vi "CalculatorMain.vi"(0 "Operations Combo Box":string(combo)="Add", 1 "Load":bool, 5 "Add":bool, 7 "Delete":bool, 9 "Save":bool, 11 "error in":errorcluster, 12 "Tree":string(tree)) -> (15 "error out":errorcluster)   [LabVIEW 2023]
doc: "This is a simple calculator which can perform basic arithmetic operations like add, subtract, multiply and divide."
uses:
  Typedef/ClassClusters.ctl
  Arithmetic/Arithmetic.lvclass
  Typedef/InstancesArray.ctl
  Typedef/DVRcluster.ctl
  Typedef/DVRInstances.ctl
  Typedef/OperationsCluster.ctl
  Typedef/QueueOperations.ctl
  e65ca531-41e1-4409-bf9f-30391f5100e7.vi
  e245d3c5-e7f7-4b04-94a4-c7f52ab5977d.vi
  <vilib>/Utility/xml.llb/Write to XML File(string).vi
  <vilib>/Utility/xml.llb/Read From XML File(array).vi
panel:
  # "CALCULATOR"
  # "INSTRUCTIONS\n\n1. Run the VI.\n2. Choose the operations to perform from the Operations Combo Box.\n3. Press ADD to display once instance of the operations in the Tree.\n4. Press any instances in the tree to load that particular operations in \n    the subpanel.\n5. In the Sub-panel enter the inputs and press CALCULATE to get the \n     output.\n6. Press SAVE to save the operations data in the XML file.\n7. Press LOAD to retrive the save data from the XML, and press the saved\n    instance in the tree to display in the subpanel.\n8. Select any instance and press DELETE to reove from the tree.\n9. Close the Front panel to abort the VI."
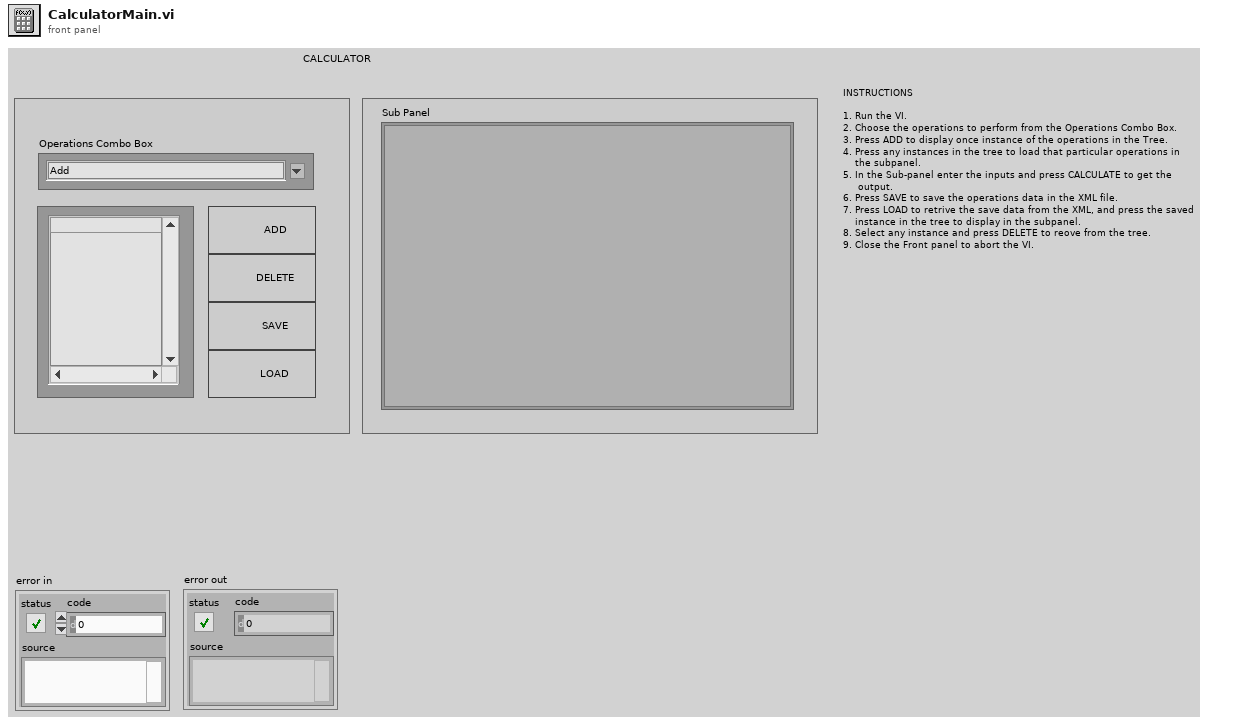
[diagram p1: front panel]
types:
  T1 = typedef "QueueOperations.ctl" = enum16{"Create", "Enqueue", "Enqueue N elements", "Dequeue", "Flush", "Release"}
  T2 = typedef "ClassClusters.ctl" = cluster{"Check":bool, "Combo Box":string, "Add":bool, "Delete":bool, "Path":path, "Tag":string, "Operation data":refnum<class "Arithmetic.lvclass">, "Instances Array":T3[], "XML path":path, "DVR":T4, "Operations Data":T6, "Saved Instances":string[], "Saves Instances String":string, "Saved Instances Path":path, "Class Path":path}
  T3 = typedef "InstancesArray.ctl" = cluster{"Tag":string, "Operation data":refnum<class "Arithmetic.lvclass">}
  T4 = typedef "DVRcluster.ctl" = cluster{"data value reference out":refnum<data-value>, "Operation Data DVR":refnum<data-value>, "Instances Array DVR":T5[]}
  T5 = typedef "DVRInstances.ctl" = cluster{"Operation Data DVR":refnum<data-value>, "Tag":string}
  T6 = typedef "OperationsCluster.ctl" = cluster{"A":dbl, "B":dbl, "C":dbl}
  T7 = typedef "LVPoint32TypeDef.ctl" = cluster{"Horizontal":i32, "Vertical":i32}
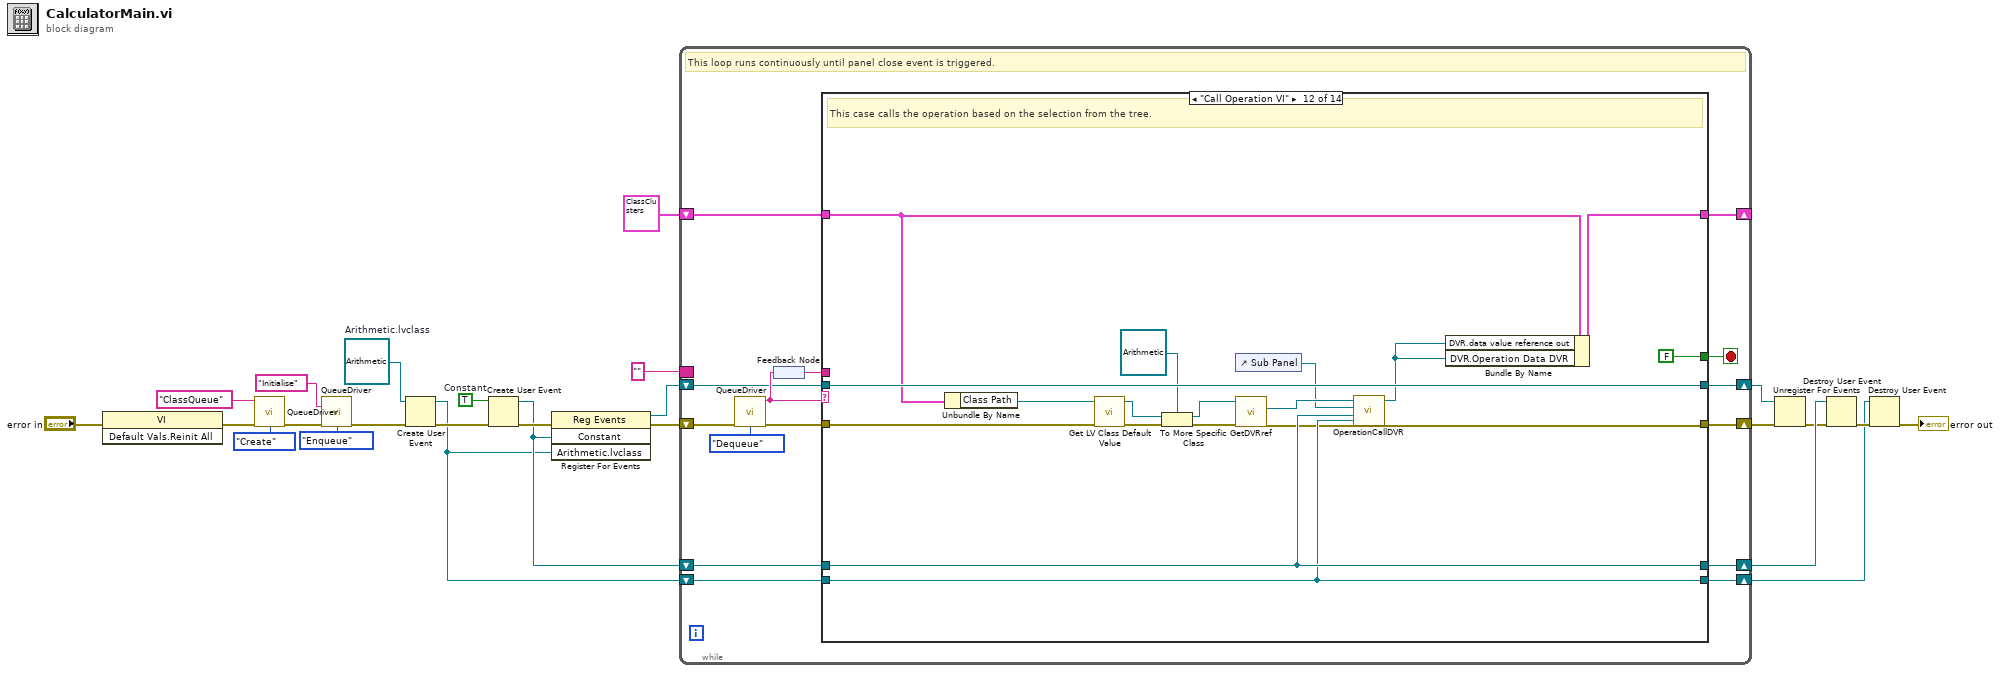
[diagram p0: block diagram]
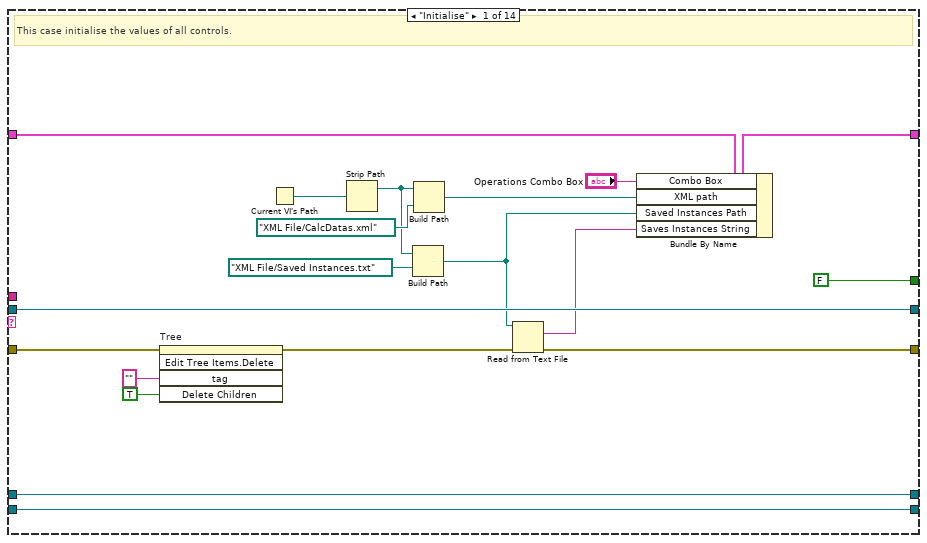
[diagram p2: hidden frame]
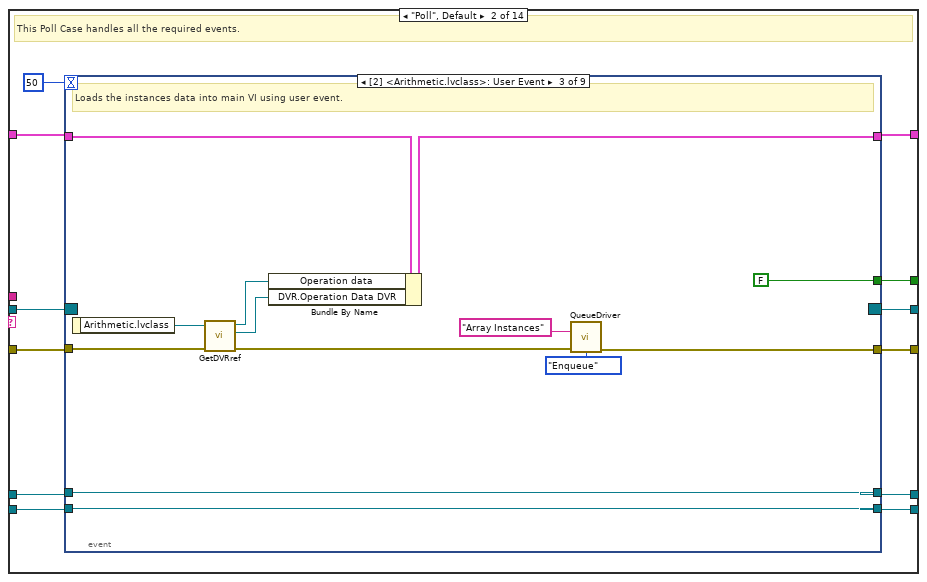
[diagram p3: hidden frame]
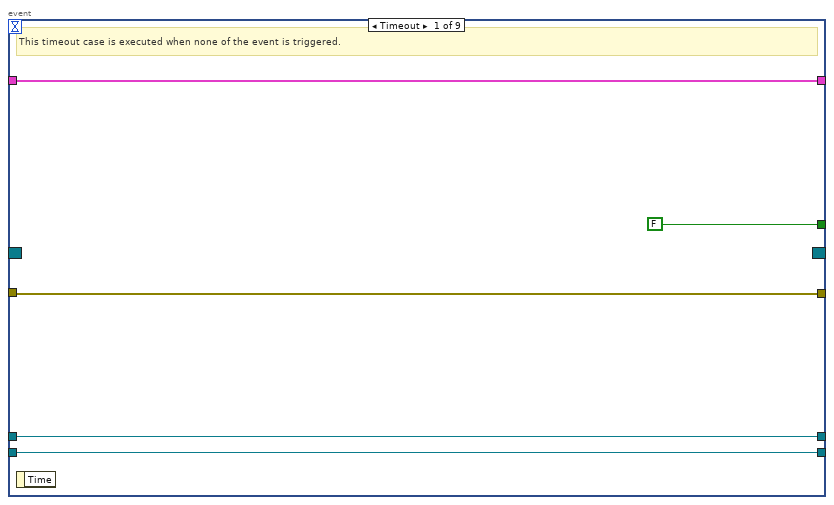
[diagram p4: hidden frame]
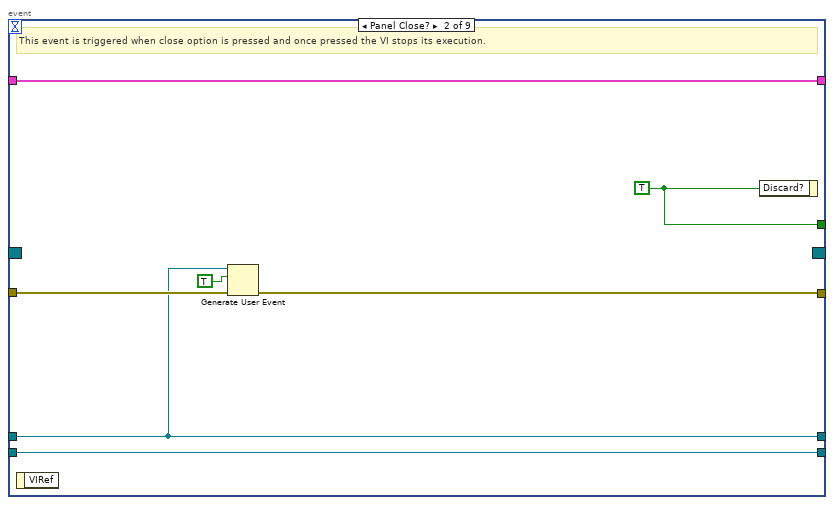
[diagram p5: hidden frame]
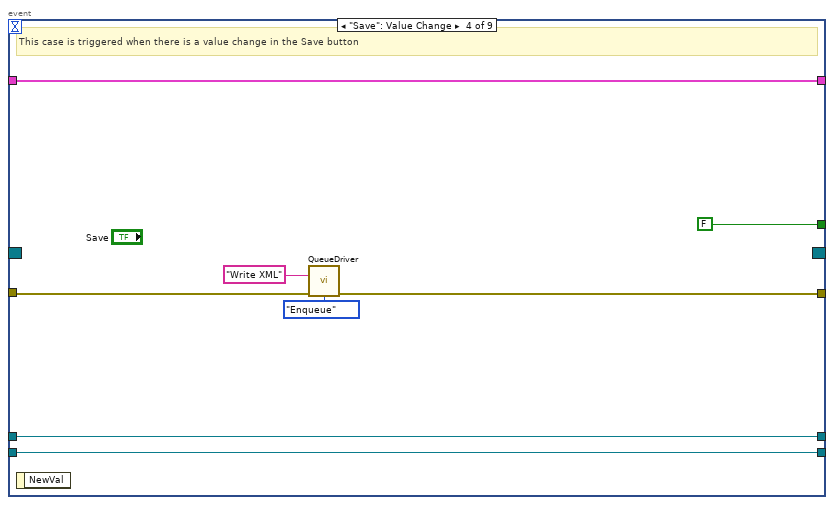
[diagram p6: hidden frame]
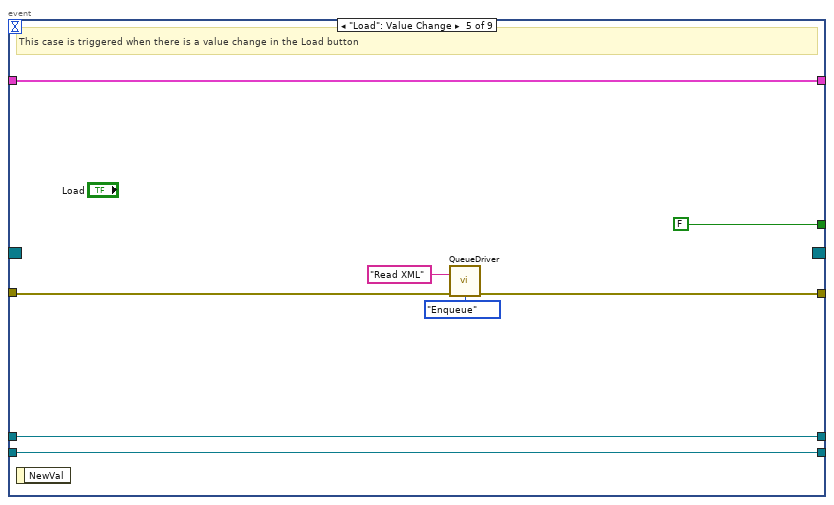
[diagram p7: hidden frame]
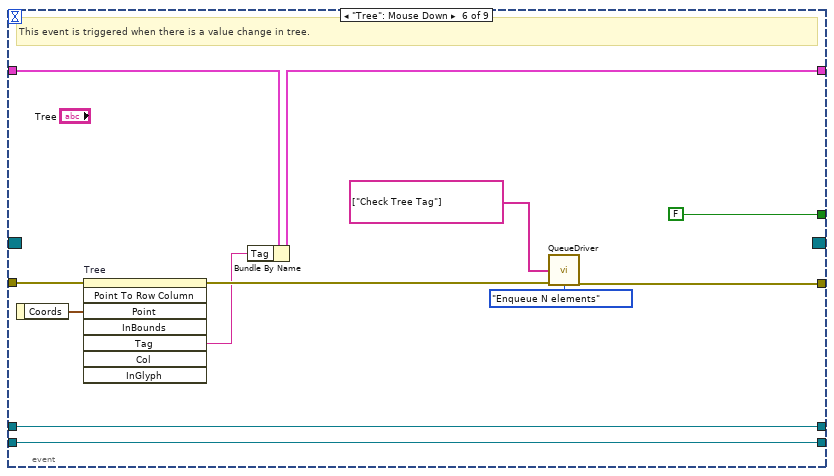
[diagram p8: hidden frame]
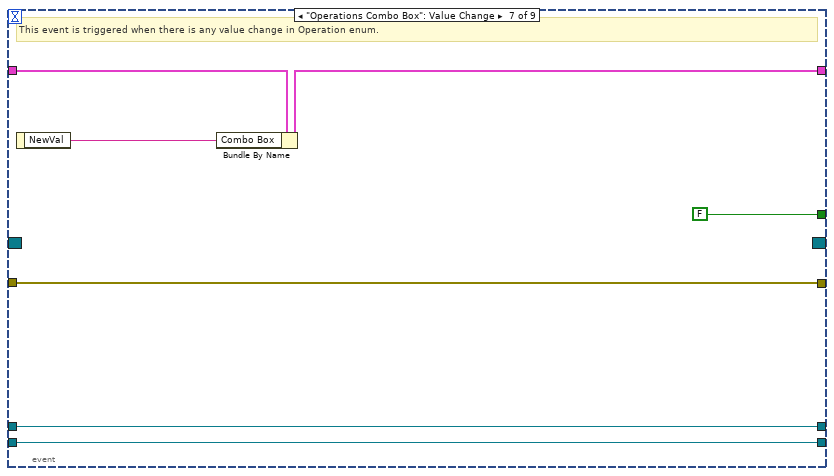
[diagram p9: hidden frame]
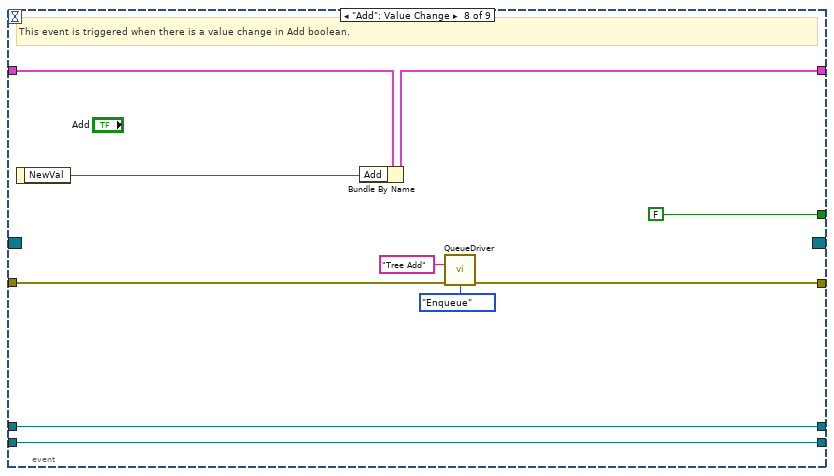
[diagram p10: hidden frame]
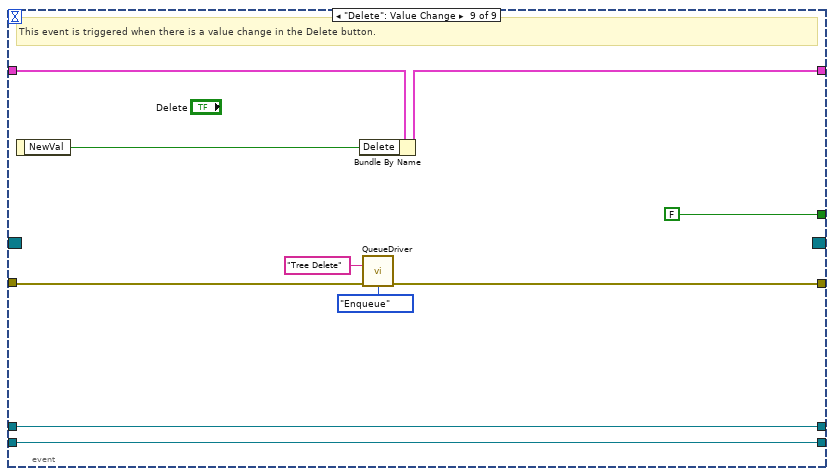
[diagram p11: hidden frame]
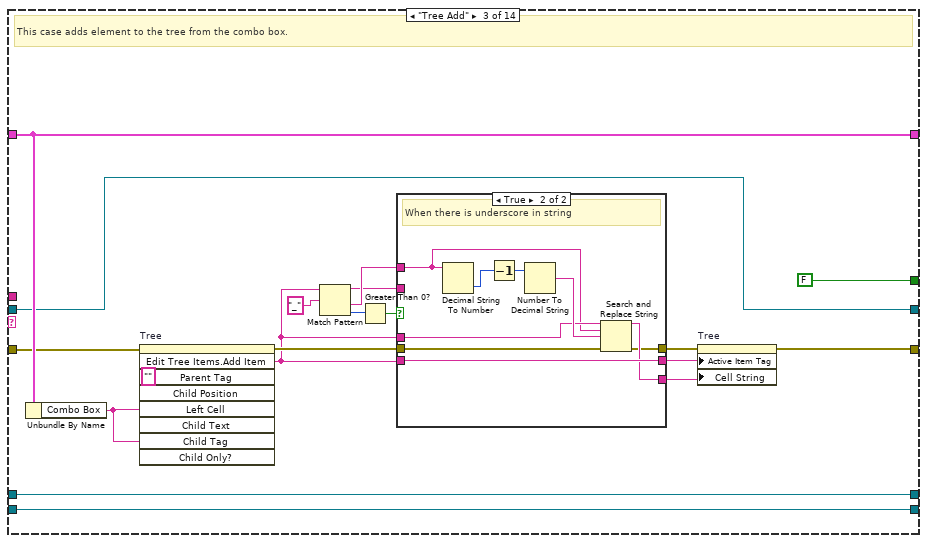
[diagram p12: hidden frame]
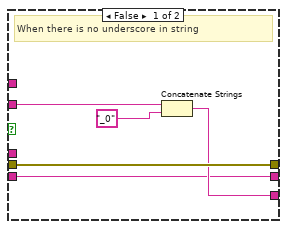
[diagram p13: hidden frame]
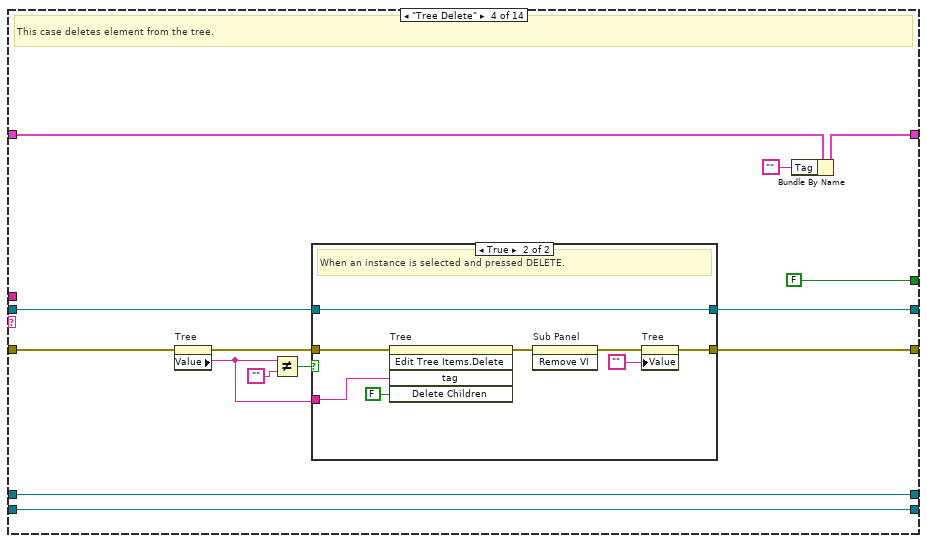
[diagram p14: hidden frame]
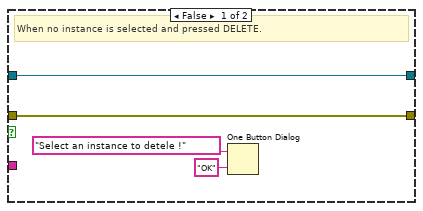
[diagram p15: hidden frame]
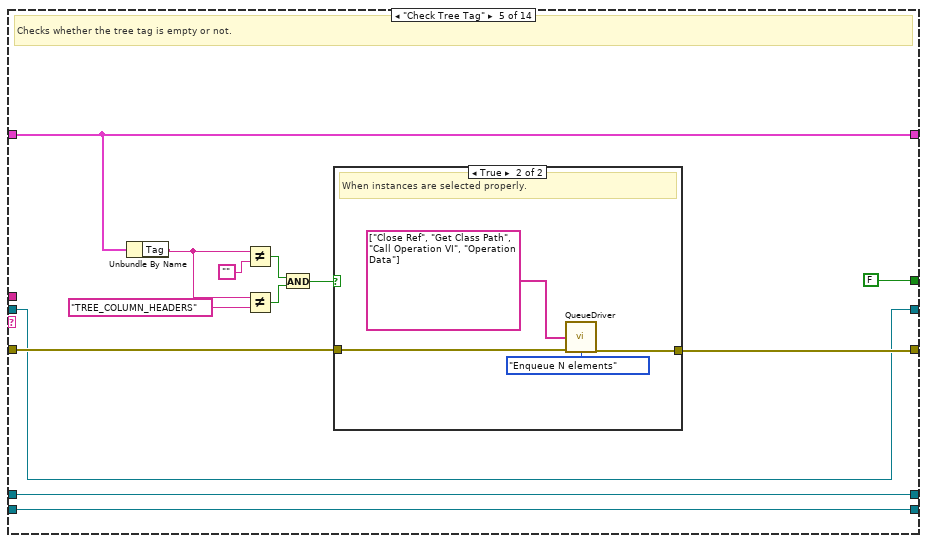
[diagram p16: hidden frame]
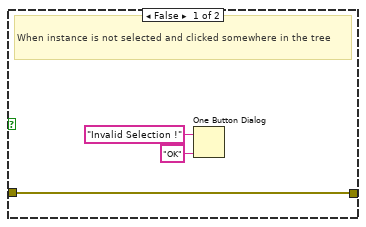
[diagram p17: hidden frame]
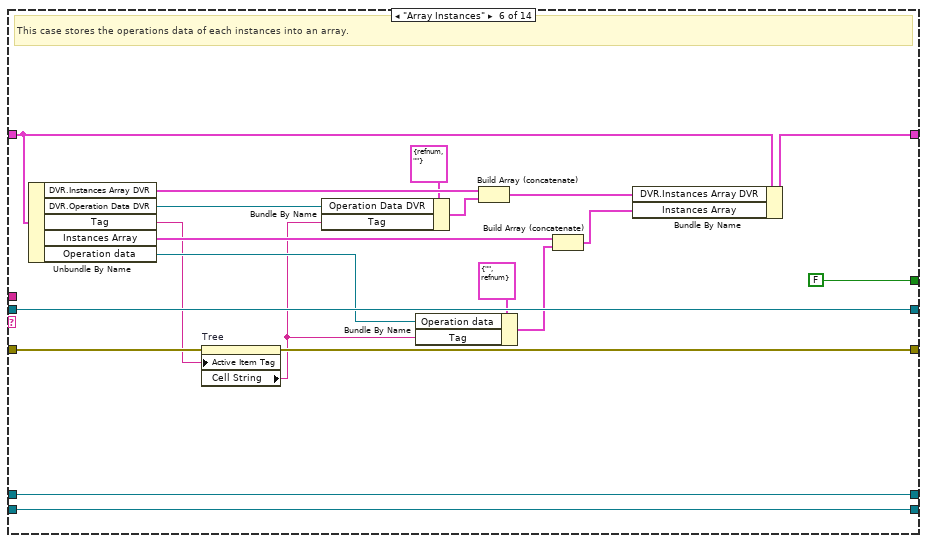
[diagram p18: hidden frame]
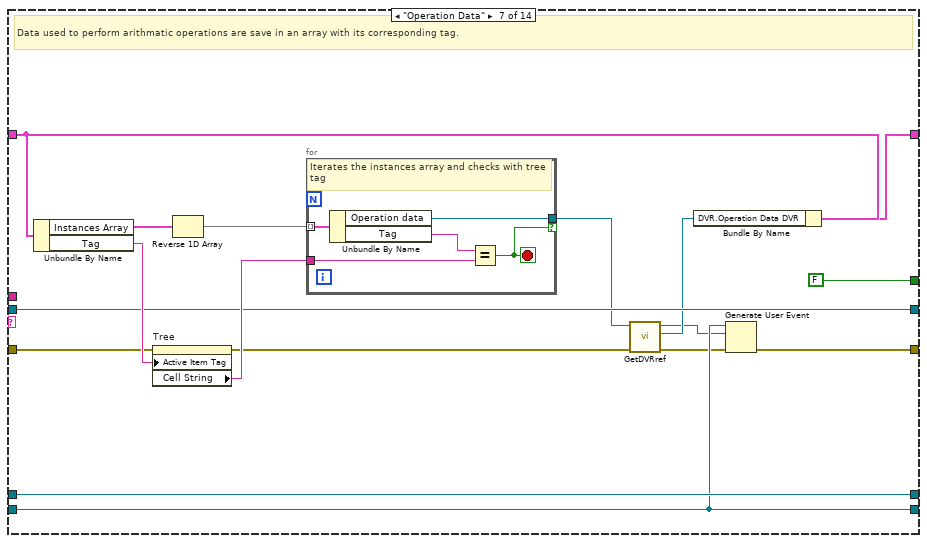
[diagram p19: hidden frame]
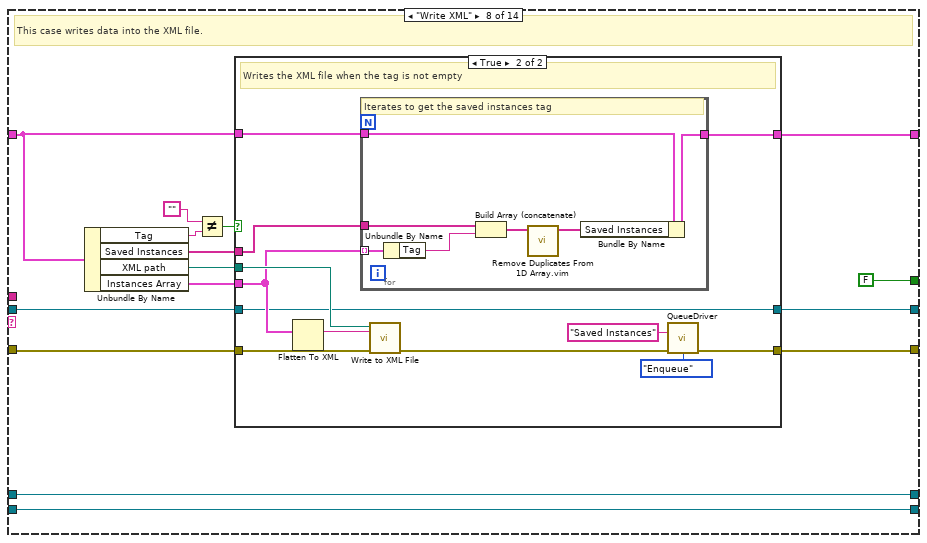
[diagram p20: hidden frame]
diagram:
  w5 = refnum<class "Arithmetic.lvclass"> refnum  # Arithmetic.lvclass
  w12 = TRUE  # Constant
  n1 = invoke class="VI" method="Default Vals.Reinit All"(error in="error in") -> (error out=w17:errorcluster)  [unwired: 2 in, 2 out]
  n2 = call "QueueDriver.vi"("Queue Name"="ClassQueue", "error in"=w17, "Queue Operations"=QueueOperations."Create") -> ("error out"=w24:errorcluster)  [unwired: 11 in, 1 out]
  n3 = call "QueueDriver.vi"("Enqueue State"="Initialise", "error in"=w24, "Queue Operations"=QueueOperations."Enqueue") -> ("error out"=w16:errorcluster)  [unwired: 11 in, 1 out]
  n4 = Create User Event(user event datatype=w5, error in=w16) -> (user event=w1:refnum<user-event>, error out=w15:errorcluster)
  n5 = Create User Event(user event datatype=w12, error in=w15) -> (user event=w10:refnum<user-event>, error out=w14:errorcluster)
  n6 = register-events(error in=w14, w10, w1) -> (reference out=w11:refnum<event-registration>, error out=w13:errorcluster)  [unwired: 1 in]
  n7 = while {
    shift-right: [w39] -> _
    shift-left: T2 {"Check"=FALSE, "Combo Box"="", "Add"=FALSE, "Delete"=FALSE, "Path"=path "", "Tag"="", "Operation data"=refnum, "Instances Array"=[], "XML path"=path "", "DVR"={"data value reference out"=refnum, "Operation Data DVR"=refnum, "Instances Array DVR"=[]}, "Operations Data"={"A"=0.0, "B"=0.0, "C"=0.0}, "Saved Instances"=[], "Saves Instances String"="", "Saved Instances Path"=path "", "Class Path"=path ""} -> [w40]
    shift-right: [w35] -> w4
    shift-left: w13 -> [w38]
    border: "" ("Dequeue State") -> [_]
    shift-right: [w26] -> w2
    shift-left: w11 -> [w29]
    shift-right: [w28] -> w8
    shift-left: w10 -> [w31]
    shift-right: [w27] -> w6
    shift-left: w1 -> [w30]
    stop <- w32 stop-if-true
    # "This loop runs continuously until panel close event is triggered."
    n8 = call "QueueDriver.vi"("error in"=w38, "Queue Operations"=QueueOperations."Dequeue") -> ("Dequeue State"=w34:string, "error out"=w37:errorcluster)  [unwired: 12 in]
    n9 = feedback #1() -> (w33:string)
    n10 = feedback-in #1(w34) -> ()
    n11 = case shown="\"Call Operation VI\"" w34 {
      tunnel: w40 -> [w59 w71 w169 w197 w220 w249 w261 w280 w325 w351 w379 w399 w408 w435]
      tunnel: [w58 w70 w169 w186 w220 w246 w259 w279 w321 w351 w372 w388 w408 w435] -> w39
      tunnel: w37 -> [w55 w67 w168 w196 w219 w247 w263 w284 w326 w350 w382 w400 w407 w425]
      tunnel: [w45 w69 w163 w187 w218 w242 w260 w278 w315 w349 w376 w389 w406 w426] -> w35
      tunnel: w33 -> [_ _ _ _ _ _ _ _ _ _ _ _ _ w424]
      tunnel: [FALSE ("Check") w66 FALSE ("Check") FALSE ("Check") FALSE ("Check") FALSE ("Check") FALSE ("Check") FALSE ("Check") FALSE ("Check") FALSE ("Check") FALSE ("Check") FALSE ("Check") FALSE ("Check") w420] -> w32
      tunnel: w31 -> [w53 w65 w154 w193 w222 w241 w258 w286 w320 w353 w385 w391 w411 w421]
      tunnel: w30 -> [w54 w62 w155 w194 w221 w240 w257 w285 w319 w352 w384 w390 w410 w422]
      tunnel: w29 -> [w52 w64 w152 w189 w211 w239 w256 w274 w316 w345 w377 w401 w405 w419]
      tunnel: [w53 w63 w154 w193 w222 w241 w258 w286 w320 w353 w385 w391 w411 w421] -> w28
      tunnel: [w54 w61 w155 w194 w221 w240 w257 w285 w319 w352 w384 w390 w410 w422] -> w27
      tunnel: [w52 w60 w152 w188 w211 w239 w256 w273 w316 w344 w377 w401 w404 w419] -> w26
      frame "Initialise" {
        # "This case initialise the values of all controls."
        n12 = invoke on="Tree" class="Tree (strict)" method="Edit Tree Items.Delete"(error in=w55, "tag"="" ("Tag"), "Delete Children"=TRUE ("Delete Children?")) -> (error out=w46:errorcluster)  [unwired: 2 in, 4 out]
        n13 = Current VI's Path() -> (path=w49:path)
        n14 = Strip Path(path=w49) -> (stripped path=w44:path)  [unwired: 1 out]
        n15 = Build Path(base path=w44, name or relative path=path "XML File/Saved Instances.txt") -> (appended path=w41:path)
        n16 = Build Path(base path=w44, name or relative path=path "XML File/CalcDatas.xml") -> (appended path=w47:path)
        n17 = Read from Text File(file (use dialog)=w41, error in=w46) -> (text=w42:string, error out=w45:errorcluster)  [unwired: 2 in, 2 out]
        n18 = Bundle By Name(cluster=w59, "Combo Box"="Operations Combo Box", "XML path"=w47, "Saved Instances Path"=w41, "Saves Instances String"=w42) -> (w58:T2)
      }
      frame "Poll", Default {
        # "This Poll Case handles all the required events."
        n19 = event shown="[2] <Arithmetic.lvclass>: User Event" {
          selector: w64 -> [_ _ _ _ _ _ _ _ _]
          dyn-events: [_ _ _ _ _ _ _ _ _] -> w60
          timeout: 50 -> [_ _ _ _ _ _ _ _ _]
          tunnel: w71 -> [w76 w83 w96 w104 w112 w124 w131 w141 w151]
          tunnel: [w76 w83 w94 w104 w112 w118 w130 w139 w149] -> w70
          tunnel: w67 -> [w75 w82 w87 w100 w108 w121 w127 w135 w145]
          tunnel: [w75 w81 w91 w99 w107 w123 w127 w134 w144] -> w69
          tunnel: [FALSE ("Check") w77 FALSE ("Check") FALSE ("Check") FALSE ("Check") FALSE ("Check") FALSE ("Check") FALSE ("Check") FALSE ("Check")] -> w66
          tunnel: w65 -> [w73 w79 w90 w98 w106 w116 w126 w133 w143]
          tunnel: [w73 w79 w90 w98 w106 w116 w126 w133 w143] -> w63
          tunnel: w62 -> [w72 w78 w89 w97 w105 w117 w125 w132 w142]
          tunnel: [w72 w78 w89 w97 w105 w117 w125 w132 w142] -> w61
          event Timeout {
            # "This timeout case is executed when none of the event is triggered."
            n20 = event-data() -> ()  [unwired: 1 in, 1 out]
          }
          event Panel Close? {
            w77 = TRUE ("Discard?")
            # "This event is triggered when close option is pressed and once pressed the VI stops its execution."
            n21 = event-data() -> ()  [unwired: 1 in, 1 out]
            n22 = Generate User Event(user event=w79, event data cluster=TRUE ("event data"), error in=w82) -> (error out=w81:errorcluster)  [unwired: 1 in, 1 out]
            n23 = event-data("Discard?"=w77) -> ()  [unwired: 1 in, 1 out]
          }
          event User Event {
            # "Loads the instances data into main VI using user event."
            n24 = event-data() -> ("Arithmetic.lvclass"=w88:refnum<class "Arithmetic.lvclass">)  [unwired: 1 in]
            n25 = call-dynamic "GetDVRref.vi"("error in (no error)"=w87, "Arithmetic in"=w88) -> ("error out"=w86:errorcluster, "data value reference"=w85:refnum<data-value>, "Arithmetic out"=w84:refnum<class "Arithmetic.lvclass">)  [unwired: 7 in]
            n26 = Bundle By Name(cluster=w96, "Operation data"=w84, "DVR.Operation Data DVR"=w85) -> (w94:T2)
            n27 = call "QueueDriver.vi"("Enqueue State"="Array Instances", "error in"=w86, "Queue Operations"=QueueOperations."Enqueue") -> ("error out"=w91:errorcluster)  [unwired: 11 in, 1 out]
          }
          event "Save": Value Change {
            # "This case is triggered when there is a value change in the Save button"
            n28 = event-data() -> ()  [unwired: 1 in, 1 out]
            n29 = call "QueueDriver.vi"("Enqueue State"="Write XML", "error in"=w100, "Queue Operations"=QueueOperations."Enqueue") -> ("error out"=w99:errorcluster)  [unwired: 11 in, 1 out]
          }
          event "Load": Value Change {
            # "This case is triggered when there is a value change in the Load button"
            n30 = event-data() -> ()  [unwired: 1 in, 1 out]
            n31 = call "QueueDriver.vi"("Enqueue State"="Read XML", "error in"=w108, "Queue Operations"=QueueOperations."Enqueue") -> ("error out"=w107:errorcluster)  [unwired: 11 in, 1 out]
          }
          event "Tree": Mouse Down {
            # "This event is triggered when there is a value change in tree."
            n32 = event-data() -> ("Coords"=w119:T7)  [unwired: 1 in]
            n33 = invoke on="Tree" class="Tree (strict)" method="Point To Row Column"(error in=w121, "Point"=w119) -> (error out=w120:errorcluster, "Tag"=w115:string)  [unwired: 6 in, 6 out]
            n34 = Bundle By Name(cluster=w124, "Tag"=w115) -> (w118:T2)
            n35 = call "QueueDriver.vi"("Array State"=string[] ["Check Tree Tag"], "error in"=w120, "Queue Operations"=QueueOperations."Enqueue N elements") -> ("error out"=w123:errorcluster)  [unwired: 11 in, 1 out]
          }
          event "Operations Combo Box": Value Change {
            # "This event is triggered when there is any value change in Operation enum."
            n36 = event-data() -> ("NewVal"=w128:string)  [unwired: 1 in]
            n37 = Bundle By Name(cluster=w131, "Combo Box"=w128) -> (w130:T2)
          }
          event "Add": Value Change {
            # "This event is triggered when there is a value change in Add boolean."
            n38 = event-data() -> ("NewVal"=w138:bool)  [unwired: 1 in]
            n39 = Bundle By Name(cluster=w141, "Add"=w138) -> (w139:T2)
            n40 = call "QueueDriver.vi"("Enqueue State"="Tree Add", "error in"=w135, "Queue Operations"=QueueOperations."Enqueue") -> ("error out"=w134:errorcluster)  [unwired: 11 in, 1 out]
          }
          event "Delete": Value Change {
            # "This event is triggered when there is a value change in the Delete button."
            n41 = event-data() -> ("NewVal"=w148:bool)  [unwired: 1 in]
            n42 = Bundle By Name(cluster=w151, "Delete"=w148) -> (w149:T2)
            n43 = call "QueueDriver.vi"("Enqueue State"="Tree Delete", "error in"=w145, "Queue Operations"=QueueOperations."Enqueue") -> ("error out"=w144:errorcluster)  [unwired: 11 in, 1 out]
          }
        }
      }
      frame "Tree Add" {
        # "This case adds element to the tree from the combo box."
        n44 = Unbundle By Name(w169) -> ("Combo Box"=w167:string)
        n45 = invoke on="Tree" class="Tree (strict)" method="Edit Tree Items.Add Item"(error in=w168, "Parent Tag"="", "Left Cell"=w167, "Child Tag"=w167) -> (error out=w165:errorcluster, "Edit Tree Items:Add Item"=w159:string)  [unwired: 5 in, 7 out]
        n46 = Match Pattern(string=w159, regular expression="_") -> (before substring=w157:string, after substring=w158:string, offset past match=w162:i32)  [unwired: 1 in, 1 out]
        n47 = Greater Than 0?(x=w162) -> (x > 0?=w161:bool)
        n48 = case shown="True" w161 {
          tunnel: w165 -> [w175 w177]
          tunnel: [w175 w176] -> w164
          tunnel: w159 -> [w172 w184]
          tunnel: [w172 w184] -> w153
          tunnel: [w173 w180] -> w160
          tunnel: w159 -> [_ w181]
          tunnel: w157 -> [w171 _]
          tunnel: w158 -> [_ w179]
          frame False {
            # "When there is no underscore in string"
            n49 = Concatenate Strings(w171, "_0" ("string")) -> (w173:string)
          }
          frame True {
            # "When there is underscore in string"
            n50 = Decimal String To Number(string=w179) -> (number=w178:i32)  [unwired: 2 in, 1 out]
            n51 = Decrement(x=w178) -> (x-1=w183:i32)
            n52 = Number To Decimal String(number=w183) -> (decimal integer string=w182:string)  [unwired: 1 in]
            n53 = Search and Replace String(input string=w181, search string=w179, replace string=w182, error in=w177) -> (result string=w180:string, error out=w176:errorcluster)  [unwired: 4 in, 2 out]
          }
        }
        n54 = property on="Tree" class="Tree (strict)"(error in=w164, "Active Item Tag"=w153, "Cell String"=w160) -> (error out=w163:errorcluster)  [unwired: 1 in, 1 out]
      }
      frame "Tree Delete" {
        # "This case deletes element from the tree."
        n55 = property on="Tree" class="Tree (strict)"(error in=w196) -> (error out=w195:errorcluster, "Value"=w190:string)  [unwired: 1 in, 1 out]
        n56 = Not Equal?(x=w190, y="") -> (x != y?=w191:bool)
        n57 = case shown="True" w191 {
          tunnel: w195 -> [w201 w210]
          tunnel: [w201 w203] -> w187
          tunnel: w190 -> [_ w208]
          tunnel: w189 -> [w202 w207]
          tunnel: [w202 w207] -> w188
          frame False {
            # "When no instance is selected and pressed DELETE."
            n58 = One Button Dialog(message="Select an instance to detele !", button name ("OK")="OK") -> ()  [unwired: 1 out]
          }
          frame True {
            # "When an instance is selected and pressed DELETE."
            n59 = invoke on="Tree" class="Tree (strict)" method="Edit Tree Items.Delete"(error in=w210, "tag"=w208, "Delete Children"=FALSE ("Delete Children?")) -> (error out=w206:errorcluster)  [unwired: 2 in, 4 out]
            n60 = invoke on="Sub Panel" class="SubPnl" method="Remove VI"(error in=w206) -> (error out=w204:errorcluster)  [unwired: 2 in, 2 out]
            n61 = property on="Tree" class="Tree (strict)"(error in=w204, "Value"="") -> (error out=w203:errorcluster)  [unwired: 1 in, 1 out]
          }
        }
        n62 = Bundle By Name(cluster=w197, "Tag"="") -> (w186:T2)
      }
      frame "Check Tree Tag" {
        # "Checks whether the tree tag is empty or not."
        n63 = Unbundle By Name(w220) -> ("Tag"=w214:string)
        n64 = Not Equal?(x=w214, y="") -> (x != y?=w217:bool)
        n65 = Not Equal?(x=w214, y="TREE_COLUMN_HEADERS") -> (x != y?=w216:bool)
        n66 = And(x=w217, y=w216) -> (x .and. y?=w212:bool)
        n67 = case shown="True" w212 {
          tunnel: [w226 w229] -> w218
          tunnel: w219 -> [w226 w228]
          frame False {
            # "When instance is not selected and clicked somewhere in the tree"
            n68 = One Button Dialog(message="Invalid Selection !", button name ("OK")="OK") -> ()  [unwired: 1 out]
          }
          frame True {
            # "When instances are selected properly."
            n69 = call "QueueDriver.vi"("Array State"=string[] ["Close Ref", "Get Class Path", "Call Operation VI", "Operation Data"], "error in"=w228, "Queue Operations"=QueueOperations."Enqueue N elements") -> ("error out"=w229:errorcluster)  [unwired: 11 in, 1 out]
          }
        }
      }
      frame "Array Instances" {
        # "This case stores the operations data of each instances into an array."
        n70 = Unbundle By Name(w249) -> ("DVR.Instances Array DVR"=w245:T5[], "DVR.Operation Data DVR"=w248:refnum<data-value>, "Tag"=w232:string, "Instances Array"=w234:T3[], "Operation data"=w236:refnum<class "Arithmetic.lvclass">)
        n71 = property on="Tree" class="Tree (strict)"(error in=w247, "Active Item Tag"=w232) -> (error out=w242:errorcluster, "Cell String"=w231:string)  [unwired: 1 in, 1 out]
        n72 = Bundle By Name(cluster=T5 {"Operation Data DVR"=refnum, "Tag"=""} ("DVR Instances"), "Operation Data DVR"=w248, "Tag"=w231) -> (w244:T5)
        n73 = Bundle By Name(cluster=T3 {"Tag"="", "Operation data"=refnum} ("Cluster"), "Operation data"=w236, "Tag"=w231) -> (w235:T3)
        n74 = Build Array (concatenate)(w245, w244) -> (w243:T5[])
        n75 = Build Array (concatenate)(w234, w235) -> (w233:T3[])
        n76 = Bundle By Name(cluster=w249, "DVR.Instances Array DVR"=w243, "Instances Array"=w233) -> (w246:T2)
      }
      frame "Operation Data" {
        # "Data used to perform arithmatic operations are save in an array with its corresponding tag."
        n77 = Unbundle By Name(w261) -> ("Instances Array"=w266:T3[], "Tag"=w264:string)
        n78 = property on="Tree" class="Tree (strict)"(error in=w263, "Active Item Tag"=w264) -> (error out=w255:errorcluster, "Cell String"=w262:string)  [unwired: 1 in, 1 out]
        n79 = Reverse 1D Array(array=w266) -> (reversed array=w265:T3[])
        n80 = for {
          tunnel: w265 -> [w272] mode=indexing
          tunnel: w262 -> [w271]
          tunnel: [w269] -> w253 if=w268
          stop <- w268 stop-if-true
          # "Iterates the instances array and checks with tree tag"
          n81 = Unbundle By Name(w272) -> ("Operation data"=w269:refnum<class "Arithmetic.lvclass">, "Tag"=w270:string)
          n82 = Equal?(x=w270, y=w271) -> (x = y?=w268:bool)
        }
        n83 = call-dynamic "GetDVRref.vi"("error in (no error)"=w255, "Arithmetic in"=w253) -> ("error out"=w254:errorcluster, "data value reference"=w252:refnum<data-value>, "Arithmetic out"=w251:refnum<class "Arithmetic.lvclass">)  [unwired: 7 in]
        n84 = Bundle By Name(cluster=w261, "DVR.Operation Data DVR"=w252) -> (w259:T2)
        n85 = Generate User Event(user event=w257, event data cluster=w251, error in=w254) -> (error out=w260:errorcluster)  [unwired: 1 in, 1 out]
      }
      frame "Write XML" {
        # "This case writes data into the XML file."
        n86 = Unbundle By Name(w280) -> ("Tag"=w276:string, "Saved Instances"=w281:string[], "XML path"=w283:path, "Instances Array"=w282:T3[])
        n87 = Not Equal?(x="", y=w276) -> (x != y?=w277:bool)
        n88 = case shown="True" w277 {
          tunnel: w284 -> [w289 w301]
          tunnel: w283 -> [_ w300]
          tunnel: w282 -> [_ w299]
          tunnel: w281 -> [_ w298]
          tunnel: w280 -> [w290 w297]
          tunnel: [w290 w296] -> w279
          tunnel: [w289 w294] -> w278
          tunnel: w274 -> [w288 w291]
          tunnel: [w288 w291] -> w273
          frame False {
            # "When tried to save without selecting an instance."
          }
          frame True {
            # "Writes the XML file when the tag is not empty"
            n89 = Flatten To XML(6:w299) -> (2:w302:string)
            n90 = for {
              tunnel: w299 -> [w309] mode=indexing
              tunnel: w298 -> [w308]
              tunnel: w297 -> [w306]
              tunnel: [w305] -> w296
              # "Iterates to get the saved instances tag"
              n91 = Unbundle By Name(w309) -> ("Tag"=w307:string)
              n92 = Build Array (concatenate)(w308, w307) -> (w304:string[])
              n93 = call "Remove Duplicates From 1D Array.vim"("array"=w304) -> ("array with duplicates removed"=w303:string[])  [unwired: 10 in]
              n94 = Bundle By Name(cluster=w306, "Saved Instances"=w303) -> (w305:T2)
            }
            n95 = call-poly <vilib>:"Write to XML File.vi"("error in (no error)"=w301, "XML Input"=w302, "XML File Path"=w300) -> ("error out"=w295:errorcluster)  [unwired: 6 in, 2 out]
            n96 = call "QueueDriver.vi"("Enqueue State"="Saved Instances", "error in"=w295, "Queue Operations"=QueueOperations."Enqueue") -> ("error out"=w294:errorcluster)  [unwired: 11 in, 1 out]
          }
        }
      }
      frame "Read XML" {
        # "This case reads data from the XML file."
        n97 = Unbundle By Name(w325) -> ("Saves Instances String"=w310:string, "Tag"=w313:string, "Instances Array"=w318:T3[], "XML path"=w324:path)
        n98 = call-poly <vilib>:"Read From XML File.vi"("error in (no error)"=w326, "XML File Path"=w324) -> ("error out"=w322:errorcluster, "XML Elements"=w323:string[])  [unwired: 7 in, 1 out]
        n99 = for {
          tunnel: w323 -> [w343] mode=indexing
          shift-right: [w341] -> w314
          shift-left: w322 -> [w342]
          tunnel: w318 -> [w340]
          tunnel: [w339] -> w317 mode=concatenating
          # "Iterates and unflattens the data from XML file"
          n100 = Unflatten From XML(xml string=w343, type=w340, error in (no error)=w342) -> (value=w339:T3[], error out=w341:errorcluster)
        }
        n101 = Not Equal?(x=w313, y="") -> (x != y?=w311:bool)
        n102 = Bundle By Name(cluster=w325, "Instances Array"=w317) -> (w321:T2)
        n103 = case shown="False" w311 {
          tunnel: [w332 w337] -> w315
          tunnel: w314 -> [w333 w335]
          tunnel: w310 -> [w328 _]
          frame False {
            # "Shows the saves instance to the user."
            n104 = Format Into String(format string="Saved Instances\n%s \n%s", error in=w333, w328, "Add and select instance in tree to load the saved data" ("message")) -> (resulting string=w330:string, error out=w332:errorcluster)  [unwired: 1 in]
            n105 = One Button Dialog(message=w330, button name ("OK")="OK") -> ()  [unwired: 1 out]
          }
          frame True {
            # "Writes the saved data in the instances"
            n106 = call "QueueDriver.vi"("Enqueue State"="Operation Data", "error in"=w335, "Queue Operations"=QueueOperations."Enqueue") -> ("error out"=w337:errorcluster)  [unwired: 11 in, 1 out]
          }
        }
      }
      frame "Saved Instances" {
        # "Saves the selected instance in a text file"
        n107 = Unbundle By Name(w351) -> ("Saved Instances"=w347:string[], "Saved Instances Path"=w348:path)
        n108 = Empty Array?(array=w347) -> (empty?=w346:bool)
        n109 = case shown="True" w346 {
          tunnel: w350 -> [w358 w368]
          tunnel: [w358 w365] -> w349
          tunnel: w348 -> [_ w361]
          tunnel: w347 -> [_ w360]
          tunnel: w345 -> [w357 w359]
          tunnel: [w357 w359] -> w344
          frame True {
            # "When no instance is selected but tried to save"
            n110 = One Button Dialog(message="Do operations in any instance and press save!!", button name ("OK")="OK") -> ()  [unwired: 1 out]
          }
          frame False {
            # "Writes the saved instance data to a text file"
            n111 = call "Remove Duplicates From 1D Array.vim"("array"=w360) -> ("array with duplicates removed"=w362:string[])  [unwired: 10 in]
            n112 = Array To Spreadsheet String(delimiter (Tab)="\r\n", array=w362, 3:"%s" ("format string")) -> (spreadsheet string=w364:string)
            n113 = Open/Create/Replace File(file path (use dialog)=w361, error in=w368, access (0:read/write)=enum16{"read/write", "read-only", "write-only"}."read/write") -> (refnum out=w367:refnum<file>, error out=w366:errorcluster)  [unwired: 3 in, 1 out]
            n114 = Write to Text File(file (use dialog)=w367, text=w364, error in=w366) -> (error out=w365:errorcluster)  [unwired: 1 in, 2 out]
          }
        }
      }
      frame "Get Class Path" {
        # "Gets the path of the selected class."
        n115 = Unbundle By Name(w379) -> ("Tag"=w381:string)
        n116 = Match Pattern(string=w381, regular expression="_") -> (before substring=w375:string)  [unwired: 1 in, 3 out]
        n117 = Format Into String(format string="..\\\\Children\\\\%s\\\\%s.lvclass", error in=w382, w375, w375) -> (resulting string=w373:string, error out=w376:errorcluster)  [unwired: 1 in]
        n118 = Current VI's Path() -> (path=w378:path)
        n119 = Build Path(base path=w378, name or relative path=w373) -> (appended path=w371:path)
        n120 = Bundle By Name(cluster=w379, "Class Path"=w371) -> (w372:T2)
      }
      frame "Call Operation VI" {
        # "This case calls the operation based on the selection from the tree."
        n121 = Unbundle By Name(w399) -> ("Class Path"=w386:path)
        n122 = call <vilib>:"Get LV Class Default Value.vi"("error in (no error)"=w400, "class path"=w386) -> ("error out"=w398:errorcluster, "object"=w397:refnum<class>)  [unwired: 8 in]
        n123 = To More Specific Class(target class=refnum<class "Arithmetic.lvclass"> refnum ("Parent Class"), reference=w397, error in=w398) -> (specific class reference=w395:refnum<class "Arithmetic.lvclass">, error out=w394:errorcluster)
        n124 = control-ref of="Sub Panel"() -> (w392:refnum<vi>)
        n125 = call-dynamic "GetDVRref.vi"("error in (no error)"=w394, "Arithmetic in"=w395) -> ("error out"=w389:errorcluster, "data value reference"=w393:refnum<data-value>)  [unwired: 7 in, 1 out]
        n126 = call "OperationCallDVR.vi"("event source"=w390, "user event out"=w391, "Sub Panel"=w392, "data value reference in"=w393) -> ("data value reference out"=w387:refnum<data-value>)  [unwired: 7 in]
        n127 = Bundle By Name(cluster=w399, "DVR.data value reference out"=w387, "DVR.Operation Data DVR"=w387) -> (w388:T2)
      }
      frame "Close Ref" {
        # "Closes the DVR reference."
        n128 = First Call?() -> (First Call?: T/F=w403:bool)
        n129 = case shown="False" w403 {
          tunnel: w408 -> [_ w418]
          tunnel: w407 -> [w413 w417]
          tunnel: [w413 w415] -> w406
          tunnel: w405 -> [w412 w414]
          tunnel: [w412 w414] -> w404
          frame True {
            # "Reference is not closed in the first call"
          }
          frame False {
            # "Delete referene after first call"
            n130 = Unbundle By Name(w418) -> ("DVR.data value reference out"=w416:refnum<data-value>)
            n131 = call "CloseRefDVR.vi"("error in (no error)"=w417, "data value reference in"=w416) -> ("error out"=w415:errorcluster)  [unwired: 8 in, 1 out]
          }
        }
      }
      frame "Error" {
        # "This case handles the error."
        n132 = Unbundle By Name(w425) -> ("code"=w423:i32, "source"=w427:string)
        n133 = call <vilib>:"Clear Errors.vi"("error in (no error)"=w425, "specific error code to clear (0: all)"=w423) -> ("error out"=w431:errorcluster)  [unwired: 4 in, 1 out]
        n134 = Format Into String(format string="Error occurred in state \"%s\"!!\nError Code: %d\nError Source: %s\n\nDo you wish to continue?", error in=w431, w424, w423, w427) -> (resulting string=w432:string, error out=w434:errorcluster)  [unwired: 1 in]
        n135 = Two Button Dialog(message=w432, 1:"Exit" ("F button name (\"Cancel\")"), 2:"Continue" ("T button name (\"OK\")")) -> (T button?=w433:bool)
        n136 = case shown="False" w433 {
          tunnel: w434 -> [w437 w439]
          tunnel: [w437 w439] -> w426
          tunnel: [TRUE ("Check") FALSE ("Check")] -> w420
          frame False {
            # "Exit"
          }
          frame True {
            # "Continue"
          }
        }
      }
    }
  }
  n137 = Unregister For Events(event registration refnum=w2, error in=w4) -> (error out=w3:errorcluster)
  n138 = Destroy User Event(user event=w8, error in=w3) -> (error out=w9:errorcluster)
  n139 = Destroy User Event(user event=w6, error in=w9) -> (error out=→"error out":errorcluster)
